vi "Build Parameters.vi"() -> (2 "Scenarios":T1(array[cluster]))   [LabVIEW 2020, in "API Pass Output.lvclass"]
doc: "This helper function simplifies the syntax of creating parameters."
uses:
  API Pass Output.lvclass
  <vilib>/Astemes/LUnit Parameterized/Parameterized Test Case/Parameterized Test Case.lvclass
  C:/Program Files/National Instruments/LabVIEW 2026/vi.lib/Astemes/LUnit Parameterized/Parameterized Test Case/Parameterized Test Case.lvclass
  API Pass Output.lvclass/API Pass Output.ctl
  Parameters.ctl
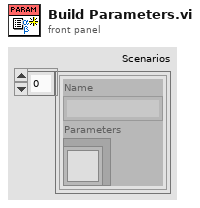
[diagram p1: front panel]
types:
  T1 = cluster{"Name":string, "Parameters":refnum<class "Parameterized Test Case.lvclass">}[]
  T2 = typedef "API Pass Output.lvclass/Parameters.ctl" = cluster{"Path":path, "Pass?":bool}
  T3 = cluster{"Scenario":string, "Parameters":refnum<class "API Pass Output.lvclass">}
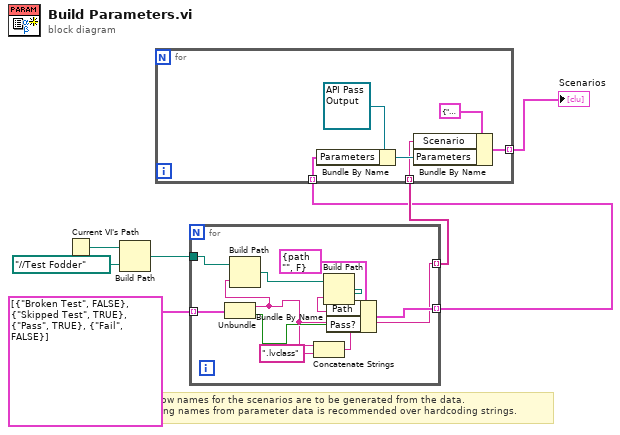
[diagram p0: block diagram]
diagram:
  # "Modify how names for the scenarios are to be generated from the data.\nGenerating names from parameter data is recommended over hardcoding strings."
  n1 = Current VI's Path() -> (path=w6:path)
  n2 = Build Path(base path=w6, name or relative path=path "../../Test Fodder") -> (appended path=w4:path)
  n3 = for {
    tunnel: w4 -> [w12]
    tunnel: cluster{string, bool}[] [{"Broken Test", FALSE}, {"Skipped Test", TRUE}, {"Pass", TRUE}, {"Fail", FALSE}] -> [w17] mode=indexing
    tunnel: [w11] -> w2 mode=indexing
    tunnel: [w15] -> w1 mode=indexing
    n4 = Unbundle(w17) -> (w11:string, w14:bool)
    n5 = Build Path(base path=w12, name or relative path=w11) -> (appended path=w10:path)
    n6 = Concatenate Strings(w11, ".lvclass" ("string")) -> (w9:string)
    n7 = Build Path(base path=w10, name or relative path=w9) -> (appended path=w8:path)
    n8 = Bundle By Name(cluster=T2 {"Path"=path "", "Pass?"=FALSE} ("Parameters"), "Path"=w8, "Pass?"=w14) -> (w15:T2)
  }
  n9 = for {
    tunnel: [w21] -> w7 mode=indexing
    tunnel: w2 -> [w19] mode=indexing
    tunnel: w1 -> [w18] mode=indexing
    n10 = Bundle By Name(cluster=refnum<class "API Pass Output.lvclass"> refnum ("Parameters"), "Parameters"=w18) -> (w22:refnum<class "API Pass Output.lvclass">)
    n11 = Bundle By Name(cluster=T3 {"Scenario"="", "Parameters"=refnum}, "Scenario"=w19, "Parameters"=w22) -> (w21:T3)
  }
  "Scenarios" <- w7
